vi "mClamp-newCard.vi"() -> ()   [LabVIEW 2010]
uses:
  <vilib>/express/express arith-compare/Formula/XNode/ExpressFormulaBlockNode.xnode
  <vilib>/DAQmx/write.llb/DAQmx Write (Digital Bool 1Line 1Point).vi
  <vilib>/DAQmx/read.llb/DAQmx Read.vi
  <vilib>/DAQmx/read.llb/DAQmx Read (Analog 1D Wfm NChan NSamp).vi
  <vilib>/daqmx/miscellaneous.llb/DAQmx Fill In Error Info.vi
  <vilib>/measure/madcrms.llb/Basic Averaged DC-RMS for N Chan.vi
  <vilib>/measure/NI_MAPro.lvlib
  <vilib>/Analysis/NI_AALBase.lvlib
panel:
  in  "DAQmx Physical Channel 2":tag
  in  "DAQmx Physical Channel":tag
  in  "stop":bool
  out "stopped":bool
  out "Voltage Pulse (mV)":dbl
  out "Current Step":dbl
  in  "Boolean 2":bool
  out "Plot":dynamicdata(graph)
  out "Resistance (MOhms)":dbl
  in  "LowTime":u32
  in  "HighTime":u32
  in  "Beta":bool
  out "pA noise":dbl
  out "Voltage noise":dbl
  in  "alpha":dbl
  # "100"
  # "Voltage Steps"
  # "1"
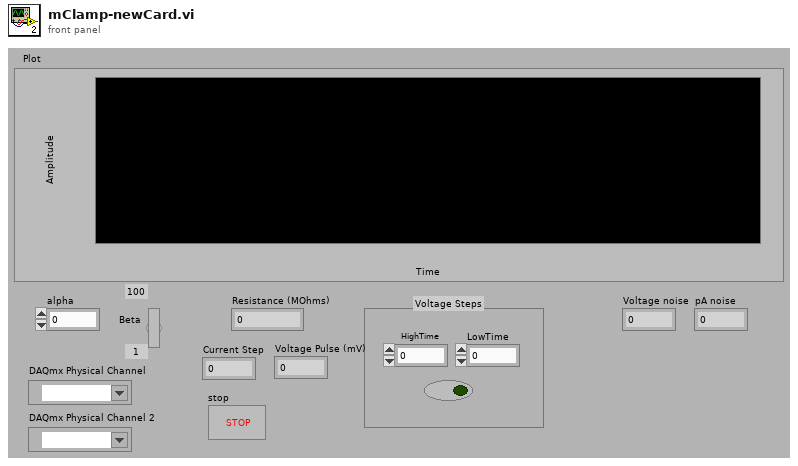
[diagram p1: front panel]
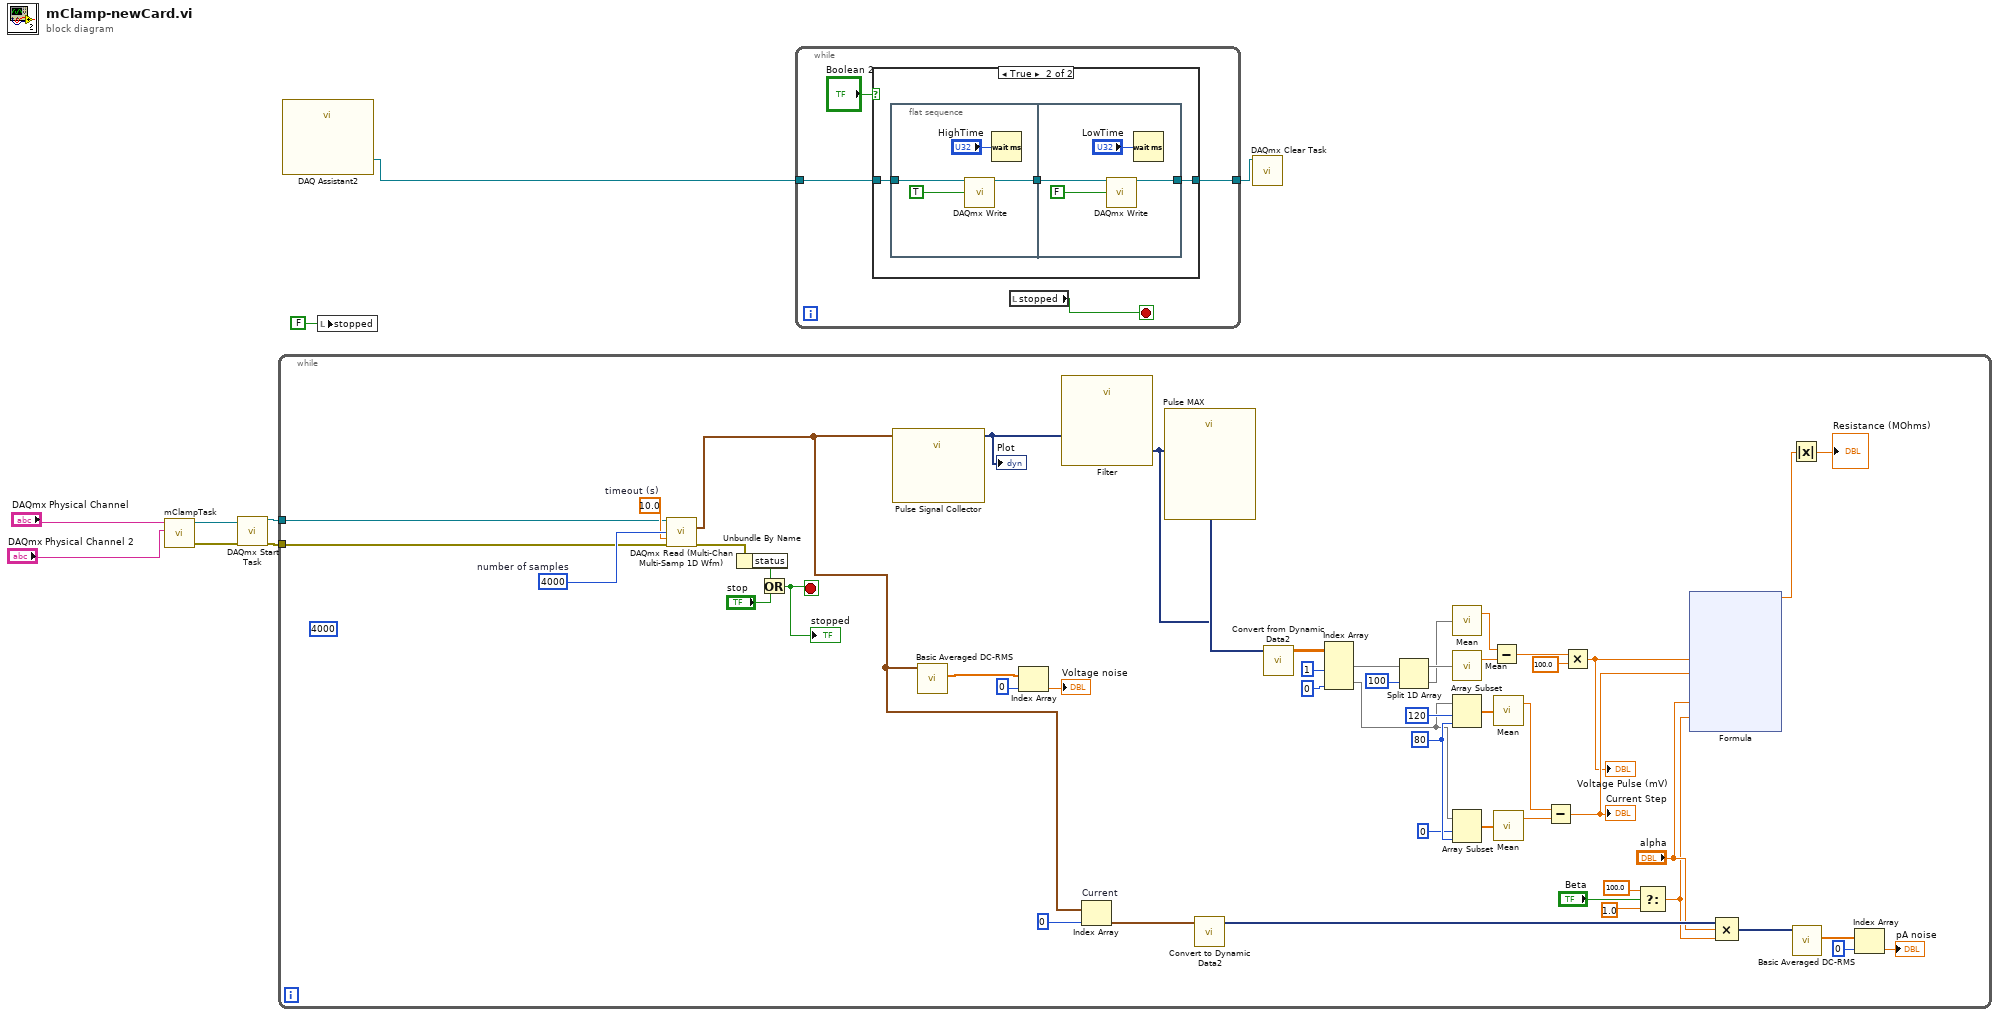
[diagram p0: block diagram]
diagram:
  n1 = call "mClampTask.vi"("physical channel 2"="DAQmx Physical Channel 2", "physical channel"="DAQmx Physical Channel") -> ("error out"=w5:errorcluster, "task out"=w6:refnum<k21>)  [unwired: 8 in]
  n2 = call <vilib>:"DAQmx Start Task.vi"("task/channels in"=w6, "error in"=w5) -> ("task out"=w4:refnum<k21>, "error out"=w3:errorcluster)  [unwired: 12 in]
  n3 = while {
    tunnel: w4 -> [w14]
    tunnel: w3 -> [w15]
    stop <- w10 stop-if-true
    w16 = 10.0  # timeout (s)
    w20 = 4000  # number of samples
    (unwired) 4000 ("number of samples")
    w44 = 80 ("length")
    n4 = call-poly "DAQmx Read (Multi-Chan Multi-Samp 1D Wfm).vi"("task/channels in"=w14, "number of samples per channel"=w20, "timeout"=w16, "error in"=w15) -> ("data"=w13:waveform(dbl)[], "error out"=w19:errorcluster)  [unwired: 9 in, 1 out]
    n5 = Unbundle By Name(w19) -> ("status"=w18:bool)
    n6 = Or(x=w18, y="stop") -> (x .or. y?=w10:bool)
    "stopped" <- w10
    n7 = call "Pulse Signal Collector"("Signals"=w13) -> ("Collected Signals"=w22:dynamicdata)  [unwired: 9 in, 1 out]
    "Plot" <- w22
    n8 = call-poly <vilib>:"Basic Averaged DC-RMS.vi"("signals in"=w13) -> ("RMS values"=w12:dbl[])  [unwired: 7 in, 3 out]
    n9 = Index Array(array=w12, index=0) -> (element=→"Voltage noise":dbl)
    n10 = call "Filter"("Signal"=w22) -> ("Filtered Signal"=w21:dynamicdata)  [unwired: 9 in, 1 out]
    n11 = Index Array "Current"(array=w13, index=0) -> (element=w54:waveform(dbl))
    n12 = call "Pulse MAX"("Manual Trigger"=w21, "Signals"=w21) -> ("Triggered Signals"=w50:dynamicdata)  [unwired: 6 in, 3 out]
    n13 = call "Convert to Dynamic Data2"("Array"=w54) -> ("Dynamic Data Type"=w37:dynamicdata)  [unwired: 3 in]
    n14 = call "Convert from Dynamic Data2"("Dynamic Data Type"=w50) -> ("Array"=w32:dbl[][])  [unwired: 3 in]
    n15 = Index Array(array=w32, index (col) #1=1 ("disabled index (col)"), index (col) #2=0 ("index (col)")) -> (element #1=w29:dbl[], element #2=w26:dbl[])  [unwired: 2 in]
    n16 = Split 1D Array(array=w29, index=100) -> (first subarray=w28:dbl[], second subarray=w27:dbl[])
    n17 = call <vilib>:"Mean.vi"("X"=w27) -> ("mean"=w48:dbl)  [unwired: 1 out]
    n18 = call <vilib>:"Mean.vi"("X"=w28) -> ("mean"=w47:dbl)  [unwired: 1 out]
    n19 = Array Subset(array=w26, index=120, length=w44) -> (w42:dbl[])
    n20 = Array Subset(array=w26, index=0, length=w44) -> (w41:dbl[])
    n21 = Subtract(x=w48, y=w47) -> (x-y=w23:dbl)
    n22 = call <vilib>:"Mean.vi"("X"=w42) -> ("mean"=w40:dbl)  [unwired: 1 out]
    n23 = call <vilib>:"Mean.vi"("X"=w41) -> ("mean"=w39:dbl)  [unwired: 1 out]
    n24 = Subtract(x=w40, y=w39) -> (x-y=w53:dbl)
    "Current Step" <- w53
    n25 = Multiply(x=w23, y=100.0 ("x")) -> (x*y=w38:dbl)
    "Voltage Pulse (mV)" <- w38
    n26 = Select(t=100.0, s="Beta", f=1.0) -> (s? t:f=w24:dbl)
    n27 = xnode "Formula"("X1"=w38, "X2"=w53, "X3"="alpha", "X4"=w24) -> ("Result"=w52:dbl)  [unwired: 1 in, 1 out]
    n28 = Compound Arithmetic op=MULTIPLY(w37, "alpha", w24) -> (w36:dynamicdata)
    n29 = Absolute Value(x=w52) -> (abs(x)=→"Resistance (MOhms)":dbl)
    n30 = call-poly <vilib>:"Basic Averaged DC-RMS.vi"("signals in"=w36) -> ("RMS values"=w35:dbl[])  [unwired: 7 in, 3 out]
    n31 = Index Array(array=w35, index=0) -> (element=→"pA noise":dbl)
  }
  n32 = call "DAQ Assistant2"() -> ("task out"=w9:refnum<k21>)  [unwired: 18 in, 1 out]
  n33 = local write "stopped"(FALSE ("stopped")) -> ()
  n34 = while {
    tunnel: w9 -> [w77]
    tunnel: [w76] -> w8
    stop <- w74 stop-if-true
    n35 = case shown="True" "Boolean 2" {
      tunnel: w77 -> [w78 w80]
      tunnel: [w78 w79] -> w76
      frame False {
      }
      frame True {
        n36 = flat-sequence {
          tunnel: w80 -> [w85]
          tunnel: [w82] -> w81
          tunnel: w81 -> [w89]
          tunnel: [w86] -> w79
          frame #0 {
            n37 = call-poly <vilib>:"DAQmx Write.vi"("task/channels in"=w85, "data"=TRUE) -> ("task out"=w82:refnum<k21>)  [unwired: 11 in, 2 out]
            n38 = Wait (ms)(milliseconds to wait="HighTime") -> ()  [unwired: 1 out]
          }
          frame #1 {
            n39 = call-poly <vilib>:"DAQmx Write.vi"("task/channels in"=w89, "data"=FALSE) -> ("task out"=w86:refnum<k21>)  [unwired: 11 in, 2 out]
            n40 = Wait (ms)(milliseconds to wait="LowTime") -> ()  [unwired: 1 out]
          }
        }
      }
    }
    n41 = local read "stopped"() -> (w74:bool)
  }
  n42 = call <vilib>:"DAQmx Clear Task.vi"("task in"=w8) -> ()  [unwired: 14 in, 1 out]
